vi "UpdateSequence.vi"(8 "error in":errorcluster, 10 "Cluster IN":T1, 11 "DataLogger in":refnum<class "DataLogger.lvclass">) -> (0 "error out":errorcluster, 2 "UpdateComplete":bool, 3 "Cluster OUT":T1)   [LabVIEW 2019, in "DataLogger.lvclass"]
doc: "Update Sequence"
uses:
  DataLogger.lvclass
  <vilib>/vision/Image Controls.llb/IMAQ Image.ctl
  Common/Controls/AllPartInfo.ctl
  Controls/LocalData_DL.ctl
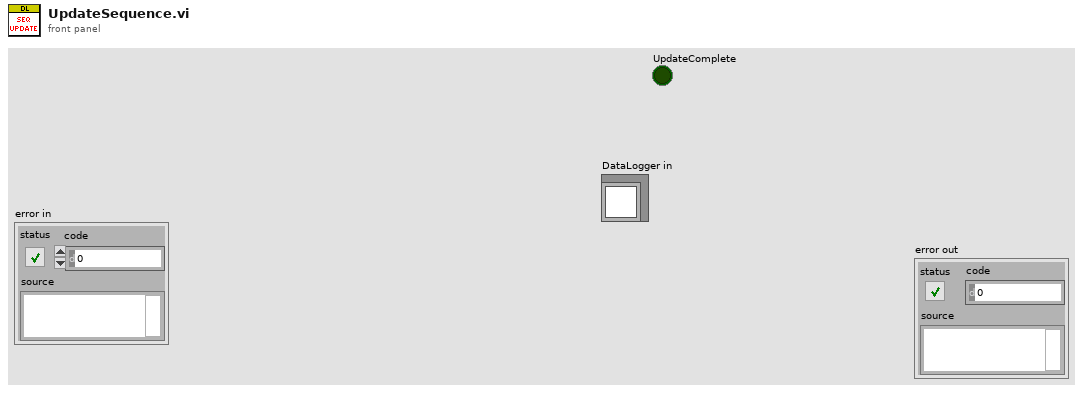
[diagram p1: front panel]
types:
  T1 = typedef "DataLogger.lvclass/LocalData_DL.ctl" = cluster{"Core":cluster{"Current VI Reference":refnum<vi>, "Close Panel on Exit?":bool}, "System Info":cluster{"System Name":string, "System ID":string, "Version":string, "Year":string, "Customer Details":cluster{"Customer Name":string, "Customer ID":string, "Location":string, "No of Shifts":u8, "Shift Details Array":cluster{"Name":string, "Timing":string}[]}, "Software Features":cluster{"IoT Enable":bool, "Datalogging Features":cluster{"Event Data":bool, "Measurement Data":bool, "Statistical Data":bool, "Reel Data":bool, "Failed Measurement Data":bool, "Failed Images":bool}, "IoT":cluster{"SMS Alert Enable":bool, "Email Alert Enable":bool}, "Popup Enable?":cluster{"Fail":bool, "Pause":bool, "Stop":bool}}}, "Part Info":cluster{"Part Name":string, "Rack ID":u8, "Initialize":bool, "StampingMc No":u64, "Operator Name":string, "ReelCount":u64, "TotalCount":u64, "Measurement Names Array":string[], "Measurement ID Array":u16[], "Spec Values Array":cluster{"LCL":dbl, "UCL":dbl, "LSL":dbl, "USL":dbl, "Nominal Value":dbl}[], "Camera Name Array":string[], "Measurement Enable/Disable Array":bool[], "Number of Measurements":i32}, "Fail Counter(For Event Details)":i32, "Event Details":cluster{"Event Name":string, "Event Time":string, "Event Reason":string, "Previous Event Name":string, "Previous Event Time":string}, "StatisticalInfo":string[][], "BatchInfo":cluster{"BatchPassCount":u64, "BatchFailCount":u64}, "Failure Details":cluster{"Fail Time Stamp":u64, "ControlPFArray":bool[], "SpecificationPFArray":dbl[], "Rack ID":u8, "Failed Image Array":T2[], "Fail Date":string, "Fail Time":string, "Fail Reason":string}, "SaveFailedImageCounter":i32, "AllPartInfoArray":T3, "Status":bool, "SpecValues(ForUpdate)":cluster{"LCL":dbl, "UCL":dbl, "LSL":dbl, "USL":dbl, "Nominal Value":dbl}, "AddSuccessfull":bool, "CurrentStateMessage":string, "IoTDetailsCounter":bool, "InitialUpdate":bool, "ResetUpdate":bool, "SetCounter":cluster{"MeasurementDetailsSetCounter":i32, "BatchDetailsSetCounter":i32, "FailureDetailsSetCounter":i32, "EventDetailsSetCounter":i32}, "IndexCounter":cluster{"MeasurementDetailsIndexCounter":i32, "BatchDetailsIndexCounter":i32, "FailureDetailsIndexCounter":i32, "EventDetailsIndexCounter":i32}, "Details2D":cluster{"MeasurementDetails(2D)":string[][], "BatchDetails(2D)":string[][], "FailureDetails(2D)":string[][], "EventDetails(2D)":string[][]}, "IDs":cluster{"Stamping McID":string, "Inspection McID":string, "BatchID":string, "FailID":string}, "Reel Info":cluster{"Reel No":u64, "Reel Start Time Stamp":u64}, "ExcelData":cluster{"StripPath":bool, "ReelCounterPerPart":i32, "FilePaths":cluster{"EventsFilePath":path, "FailFilePath":path, "ReelFilePath":path, "StatisticalFilePath":path}, "ExcelSheetCounterPerReel":cluster{"EventsSheetCounter":u32, "FailSheetCounter":u32, "StatisticalSheetCounter":u32, "ReelSheetCounter":u32}, "CreateNewExcel":cluster{"CreateNewEventsExcel":bool, "CreateNewFailExcel":bool, "CreateNewStatisticalExcel":bool, "CreateNewReelExcel":bool}, "RecordsInExcelCounter":cluster{"EventsRecordsCounter":u32, "FailRecordsCounter":u32, "ReelRecordsCounter":u32, "StatisticalRecordsCounter":u32}}, "SaveAck":cluster{"Loop1":bool, "Loop2":bool}, "Shift Statistical Info":cluster{"Shift Name":string, "Shift Timing":string, "Shift End Date":string, "Statistical Shift Data":cluster{"PartName":string, "MeasurementNames":string[], "Statistical Parameters":string[][]}[]}}
  T2 = typedef "IMAQ Image.ctl" = refnum<image>
  T3 = typedef "AllPartInfo.ctl" = cluster{"PartName":string, "NumberOfRacks":u8, "MeasurementIDsArray":u16[], "MeasurementNamesArray":string[], "SpecValuesArray":cluster{"LCL":dbl, "UCL":dbl, "LSL":dbl, "USL":dbl, "NominalValue":dbl}[]}[]
  T4 = cluster{"LCL":dbl, "UCL":dbl, "LSL":dbl, "USL":dbl, "NominalValue":dbl}[]
  T5 = cluster{"LCL":dbl, "UCL":dbl, "LSL":dbl, "USL":dbl, "Nominal Value":dbl}[]
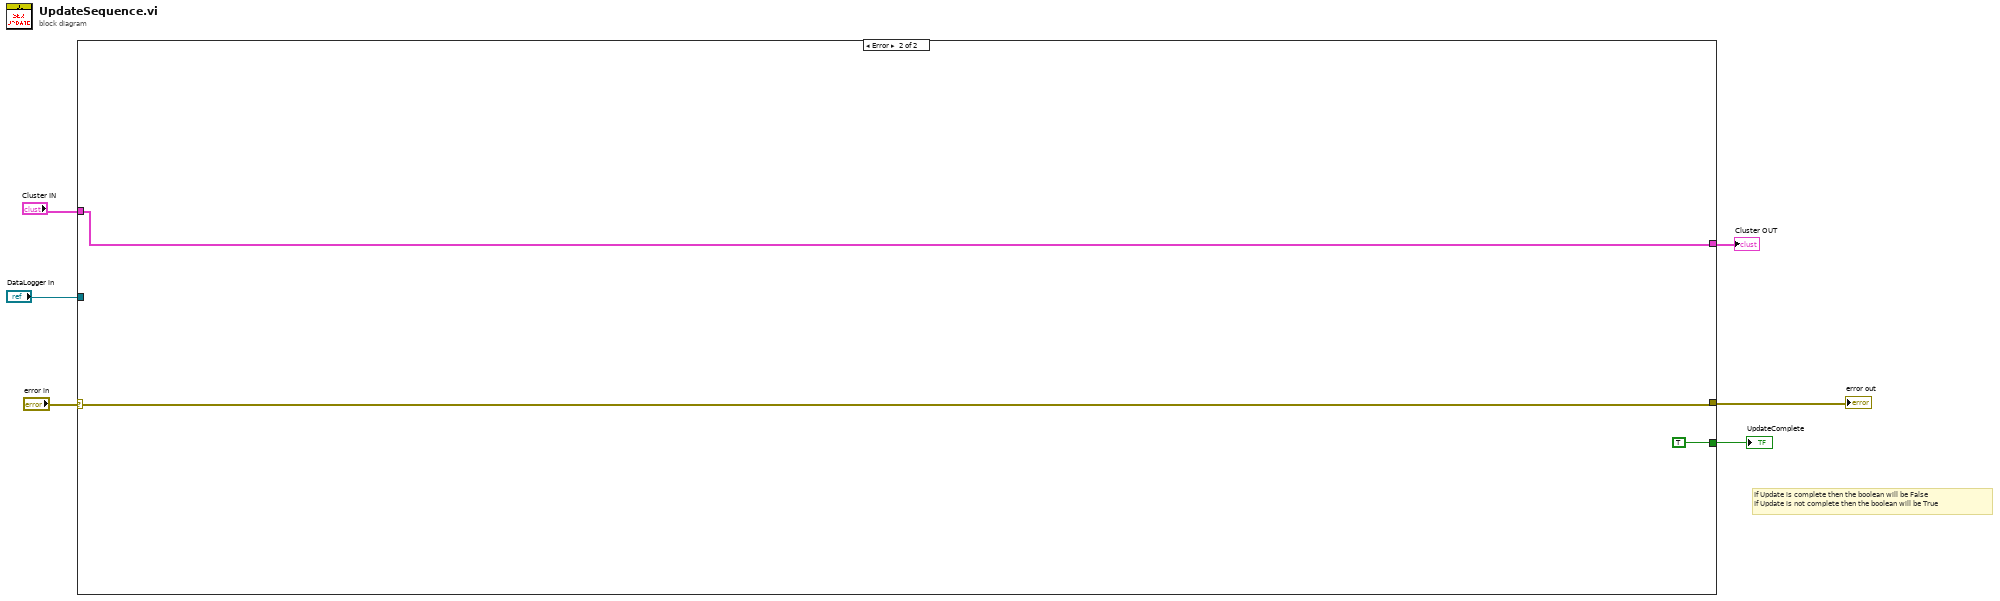
[diagram p0: block diagram]
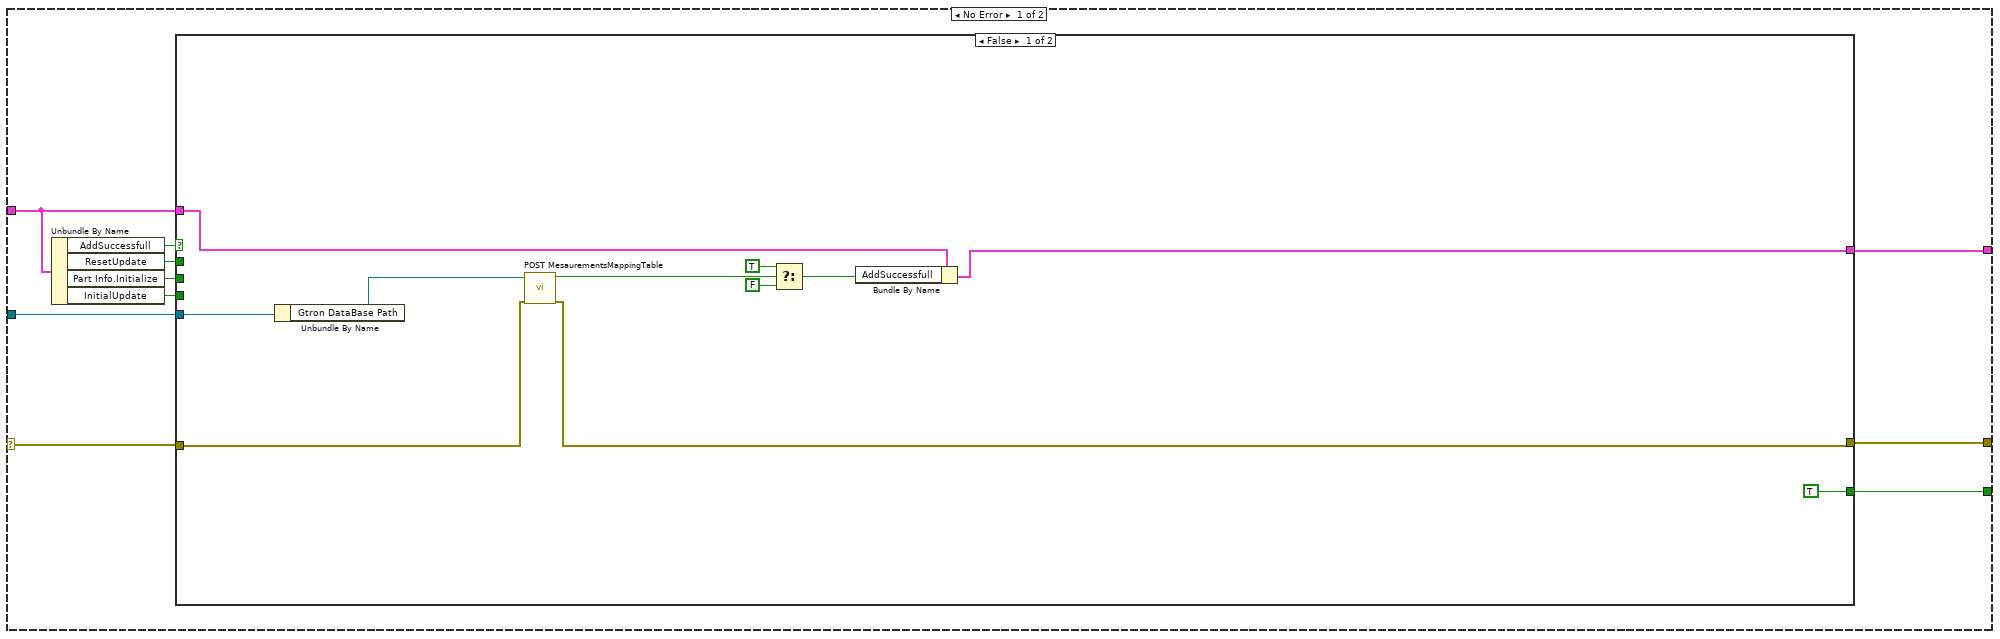
[diagram p2: hidden frame]
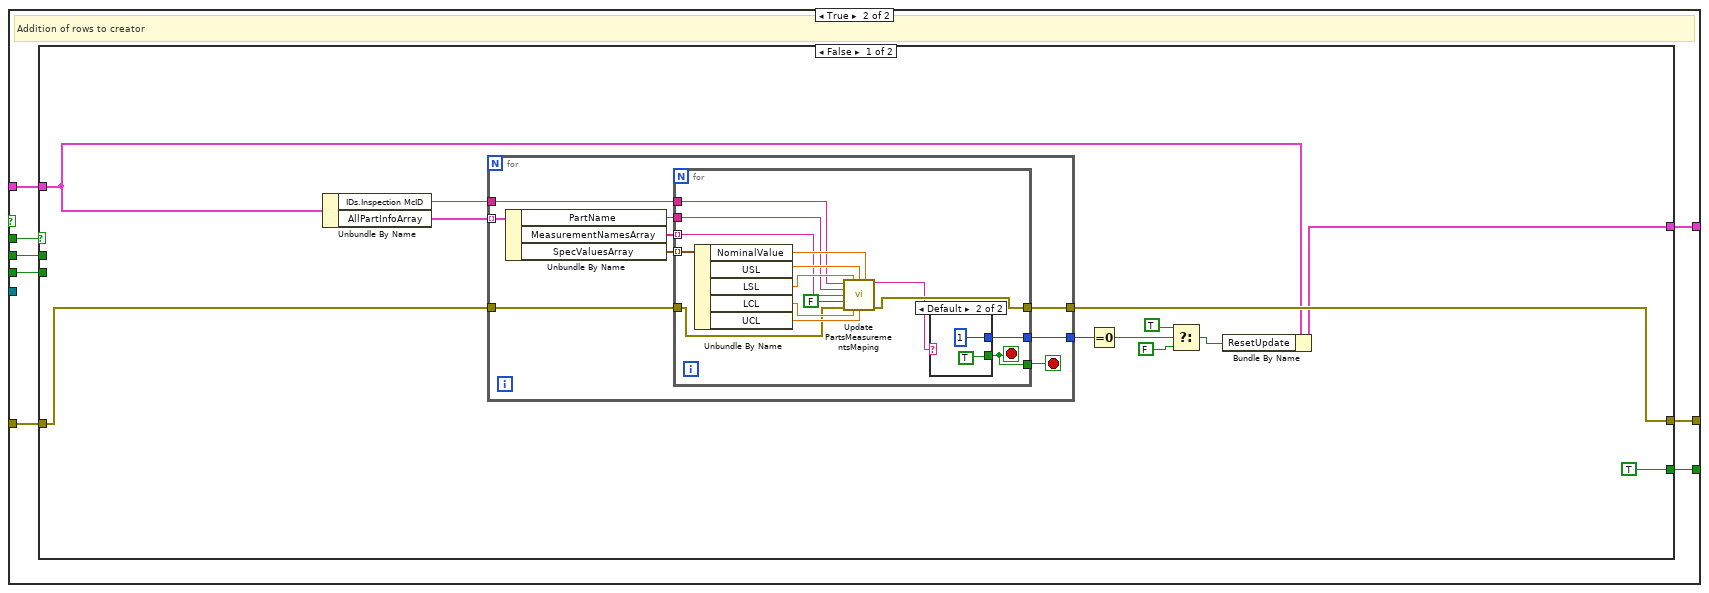
[diagram p3: hidden frame]
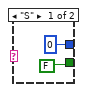
[diagram p4: hidden frame]
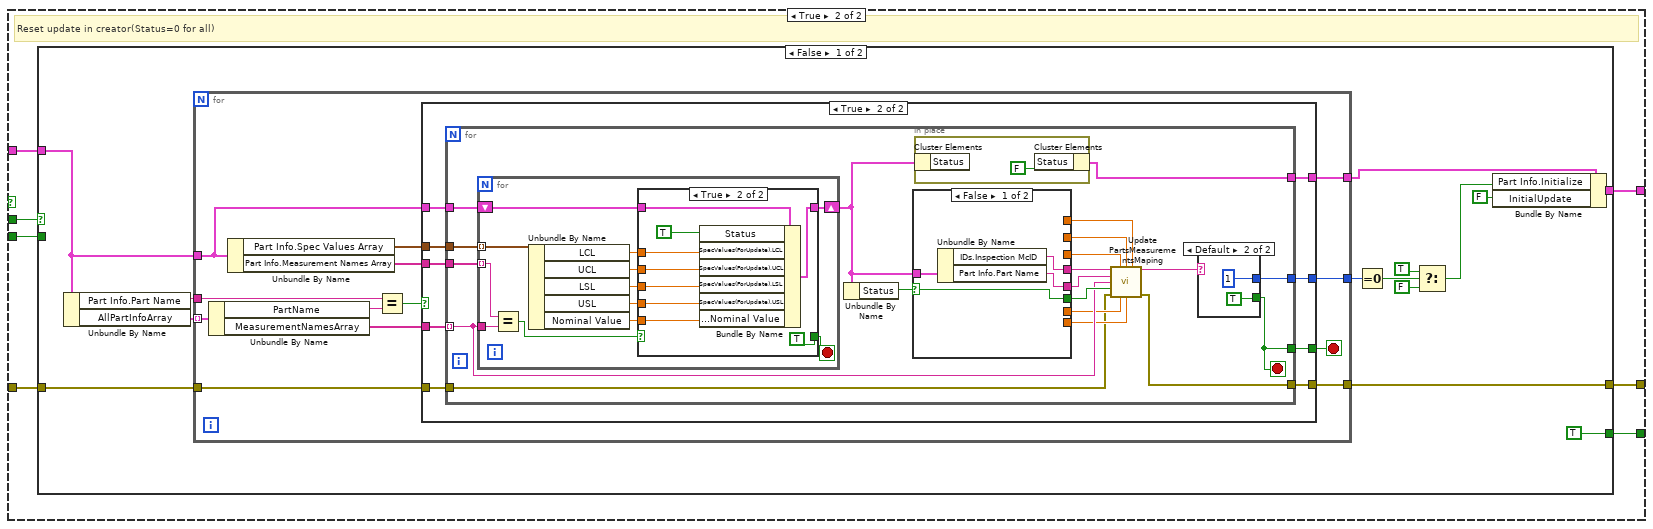
[diagram p5: hidden frame]
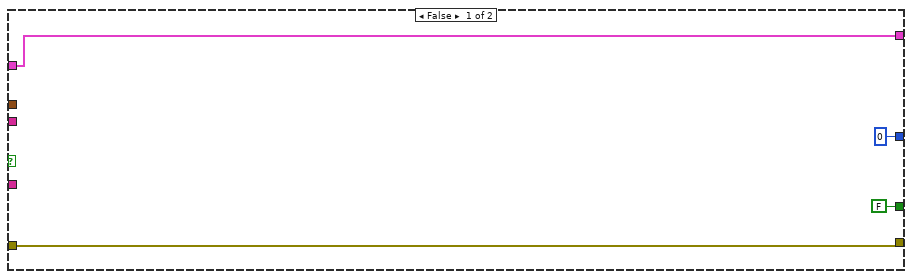
[diagram p6: hidden frame]
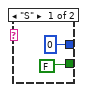
[diagram p7: hidden frame]
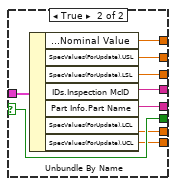
[diagram p8: hidden frame]
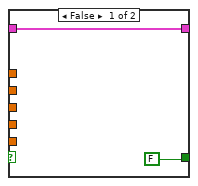
[diagram p9: hidden frame]
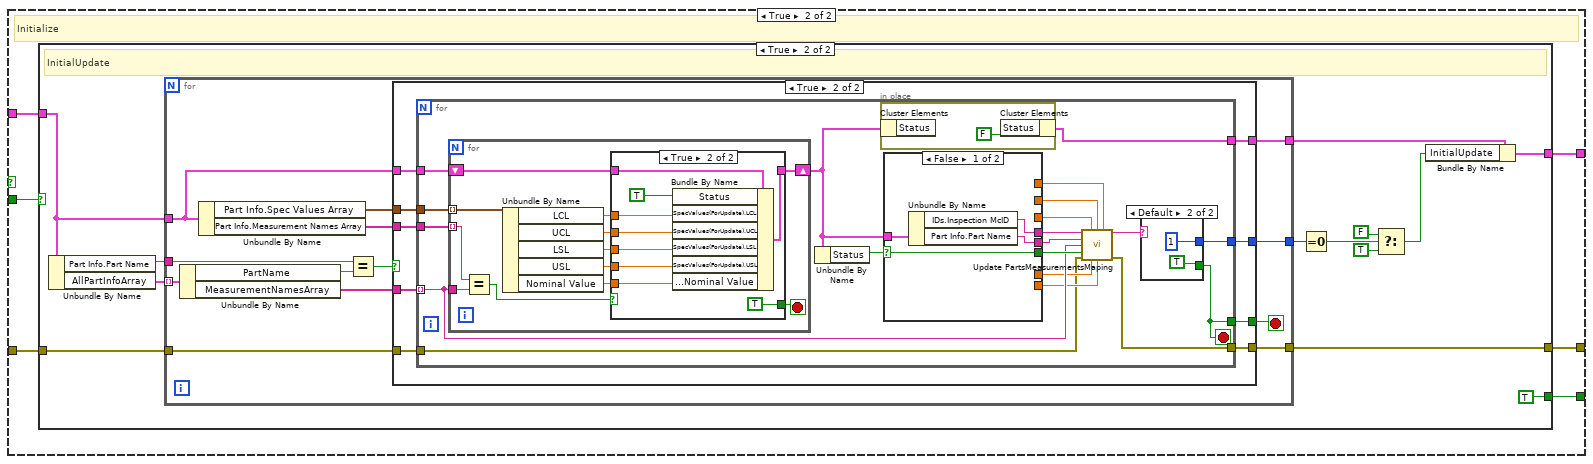
[diagram p10: hidden frame]
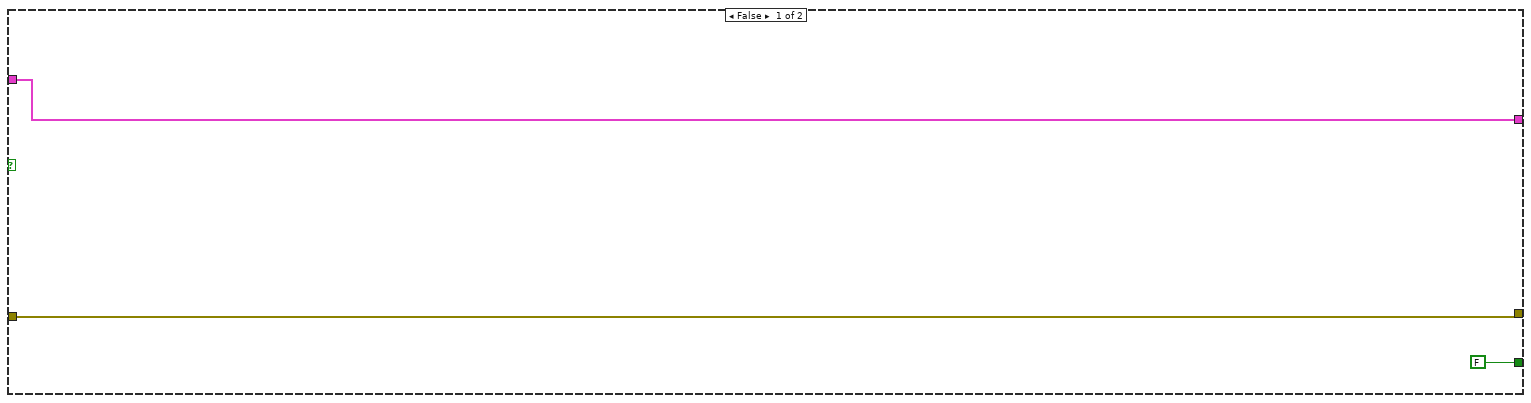
[diagram p11: hidden frame]
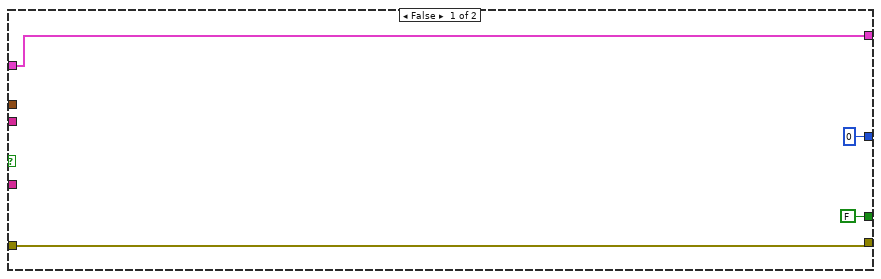
[diagram p12: hidden frame]
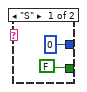
[diagram p13: hidden frame]
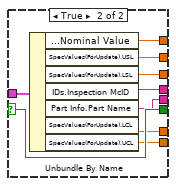
[diagram p14: hidden frame]
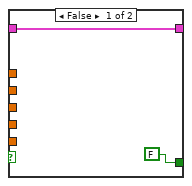
[diagram p15: hidden frame]
diagram:
  # "If Update is complete then the boolean will be False\nIf Update is not complete then the boolean will be True"
  n1 = case shown="Error" "error in" {
    selector: "error in" -> [w11 w295]
    tunnel: [w14 w295] -> w6
    tunnel: "DataLogger in" -> [w10 _]
    tunnel: "Cluster IN" -> [w9 w294]
    tunnel: [w8 w294] -> w2
    tunnel: [w7 TRUE] -> w1
    frame No Error {
      n2 = Unbundle By Name(w9) -> ("AddSuccessfull"=w15:bool, "ResetUpdate"=w16:bool, "Part Info.Initialize"=w13:bool, "InitialUpdate"=w12:bool)
      n3 = case shown="False" w15 {
        tunnel: w9 -> [w24 w35]
        tunnel: w13 -> [_ w34]
        tunnel: [w23 w33] -> w8
        tunnel: w11 -> [w19 w32]
        tunnel: [w18 w31] -> w14
        tunnel: w10 -> [w21 _]
        tunnel: w12 -> [_ w30]
        tunnel: w16 -> [_ w29]
        tunnel: [TRUE w28] -> w7
        frame False {
          n4 = Unbundle By Name(w21) -> ("Gtron DataBase Path"=w20:path)
          n5 = call "POST MesaurementsMappingTable.vi"("error in"=w19, "GTron in"=w20) -> ("error out"=w18:errorcluster, "DB is Empty?"=w22:bool)  [unwired: 8 in]
          n6 = Select(t=TRUE, s=w22, f=FALSE) -> (s? t:f=w25:bool)
          n7 = Bundle By Name(cluster=w24, "AddSuccessfull"=w25) -> (w23:T1)
        }
        frame True {
          # "Addition of rows to creator"
          n8 = case shown="False" w29 {
            tunnel: w35 -> [w40 w82]
            tunnel: w34 -> [_ w81]
            tunnel: [w41 w80] -> w33
            tunnel: w32 -> [w43 w79]
            tunnel: [w42 w78] -> w31
            tunnel: w30 -> [_ w77]
            tunnel: [TRUE w76] -> w28
            frame False {
              n9 = Unbundle By Name(w40) -> ("IDs.Inspection McID"=w39:string, "AllPartInfoArray"=w47:T3)
              n10 = for {
                tunnel: w47 -> [w56] mode=indexing
                tunnel: w43 -> [w52]
                tunnel: [w51] -> w42
                tunnel: [w49] -> w37
                tunnel: w39 -> [w48]
                stop <- w50 stop-if-true
                n11 = Unbundle By Name(w56) -> ("PartName"=w54:string, "MeasurementNamesArray"=w55:string[], "SpecValuesArray"=w53:T4)
                n12 = for {
                  tunnel: w55 -> [w66] mode=indexing
                  tunnel: w54 -> [w67]
                  tunnel: w53 -> [w71] mode=indexing
                  tunnel: w52 -> [w62]
                  tunnel: [w61] -> w51
                  tunnel: [w58] -> w50
                  tunnel: [w59] -> w49
                  tunnel: w48 -> [w57]
                  stop <- w58 stop-if-true
                  n13 = Unbundle By Name(w71) -> ("NominalValue"=w70:dbl, "USL"=w69:dbl, "LSL"=w68:dbl, "LCL"=w64:dbl, "UCL"=w63:dbl)
                  n14 = call "Update PartsMeasurementsMaping.vi"("InspectionMcId"=w57, "NewLSL"=w68, "NewUSL"=w69, "NewNominalValue"=w70, "PartName"=w67, "MeasurementName"=w66, "Status1"=FALSE ("Status"), "error in"=w62, "NewLCL"=w64, "NewUCL"=w63) -> ("Status"=w60:string, "error out"=w61:errorcluster)  [unwired: 4 in]
                  n15 = case shown="Default" w60 {
                    tunnel: [0 1] -> w59
                    tunnel: [FALSE TRUE] -> w58
                    frame "S" {
                    }
                    frame Default {
                    }
                  }
                }
              }
              n16 = Equal To 0?(x=w37) -> (x = 0?=w38:bool)
              n17 = Select(t=TRUE, s=w38, f=FALSE) -> (s? t:f=w44:bool)
              n18 = Bundle By Name(cluster=w40, "ResetUpdate"=w44) -> (w41:T1)
            }
            frame True {
              # "Reset update in creator(Status=0 for all)"
              n19 = case shown="False" w81 {
                tunnel: w82 -> [w93 w188]
                tunnel: [w94 w189] -> w80
                tunnel: w79 -> [w91 w187]
                tunnel: [w90 w186] -> w78
                tunnel: w77 -> [_ w185]
                tunnel: [TRUE w184] -> w76
                frame False {
                  n20 = Unbundle By Name(w93) -> ("Part Info.Part Name"=w95:string, "AllPartInfoArray"=w96:T3)
                  n21 = for {
                    tunnel: w96 -> [w109] mode=indexing
                    tunnel: w95 -> [w107]
                    tunnel: w93 -> [w102]
                    tunnel: [w101] -> w92
                    tunnel: w91 -> [w100]
                    tunnel: [w99] -> w90
                    tunnel: [w97] -> w85
                    stop <- w98 stop-if-true
                    n22 = Unbundle By Name(w109) -> ("PartName"=w108:string, "MeasurementNamesArray"=w105:string[])
                    n23 = Unbundle By Name(w102) -> ("Part Info.Spec Values Array"=w104:T5, "Part Info.Measurement Names Array"=w103:string[])
                    n24 = Equal?(x=w107, y=w108) -> (x = y?=w106:bool)
                    n25 = case shown="True" w106 {
                      tunnel: w105 -> [_ w122]
                      tunnel: w104 -> [_ w121]
                      tunnel: w103 -> [_ w120]
                      tunnel: w102 -> [w113 w119]
                      tunnel: [w113 w118] -> w101
                      tunnel: w100 -> [w112 w117]
                      tunnel: [w112 w116] -> w99
                      tunnel: [FALSE w115] -> w98
                      tunnel: [0 w114] -> w97
                      frame False {
                      }
                      frame True {
                        n26 = for {
                          tunnel: w122 -> [w137] mode=indexing
                          tunnel: w121 -> [w142]
                          tunnel: w120 -> [w141]
                          tunnel: w119 -> [w140]
                          tunnel: [w123] -> w118
                          tunnel: w117 -> [w129]
                          tunnel: [w128] -> w116
                          tunnel: [w126] -> w115
                          tunnel: [w125] -> w114
                          stop <- w126 stop-if-true
                          n27 = for {
                            tunnel: w142 -> [w167] mode=indexing
                            tunnel: w141 -> [w172] mode=indexing
                            tunnel: w137 -> [w171]
                            shift-right: [w168] -> w124
                            shift-left: w140 -> [w170]
                            stop <- w161 stop-if-true
                            n28 = Equal?(x=w172, y=w171) -> (x = y?=w169:bool)
                            n29 = Unbundle By Name(w167) -> ("LCL"=w162:dbl, "UCL"=w163:dbl, "LSL"=w164:dbl, "USL"=w165:dbl, "Nominal Value"=w166:dbl)
                            n30 = case shown="True" w169 {
                              tunnel: w170 -> [w174 w183]
                              tunnel: [w174 w181] -> w168
                              tunnel: w166 -> [_ w180]
                              tunnel: w165 -> [_ w179]
                              tunnel: w164 -> [_ w178]
                              tunnel: w163 -> [_ w177]
                              tunnel: w162 -> [_ w176]
                              tunnel: [FALSE TRUE] -> w161
                              frame False {
                              }
                              frame True {
                                n31 = Bundle By Name(cluster=w183, "Status"=TRUE, "SpecValues(ForUpdate).LCL"=w176, "SpecValues(ForUpdate).UCL"=w177, "SpecValues(ForUpdate).LSL"=w178, "SpecValues(ForUpdate).USL"=w179, "SpecValues(ForUpdate).Nominal Value"=w180) -> (w181:T1)
                              }
                            }
                          }
                          n32 = Unbundle By Name(w124) -> ("Status"=w139:bool)
                          n33 = case shown="False" w139 {
                            selector: w139 -> [w151 w159]
                            tunnel: w124 -> [w150 w160]
                            tunnel: [w151 w159] -> w138
                            tunnel: [_ w158] -> w136
                            tunnel: [_ w157] -> w135
                            tunnel: [_ w156] -> w134
                            tunnel: [_ w155] -> w133
                            tunnel: [_ w154] -> w132
                            tunnel: [w149 w153] -> w131
                            tunnel: [w148 w152] -> w130
                            frame False {
                              n34 = Unbundle By Name(w150) -> ("IDs.Inspection McID"=w149:string, "Part Info.Part Name"=w148:string)
                            }
                            frame True {
                              n35 = Unbundle By Name(w160) -> ("SpecValues(ForUpdate).Nominal Value"=w158:dbl, "SpecValues(ForUpdate).USL"=w157:dbl, "SpecValues(ForUpdate).LSL"=w156:dbl, "IDs.Inspection McID"=w153:string, "Part Info.Part Name"=w152:string, "SpecValues(ForUpdate).LCL"=w154:dbl, "SpecValues(ForUpdate).UCL"=w155:dbl)
                            }
                          }
                          n36 = in-place {
                            n37 = in-place-cluster #1(w124) -> ()  [unwired: 1 out]
                            n38 = in-place-cluster #1("Status"=FALSE) -> (w123:T1)
                          }
                          n39 = call "Update PartsMeasurementsMaping.vi"("InspectionMcId"=w131, "NewLSL"=w134, "NewUSL"=w135, "NewNominalValue"=w136, "PartName"=w130, "MeasurementName"=w137, "Status1"=w138, "error in"=w129, "NewLCL"=w132, "NewUCL"=w133) -> ("Status"=w127:string, "error out"=w128:errorcluster)  [unwired: 4 in]
                          n40 = case shown="Default" w127 {
                            tunnel: [0 1] -> w125
                            tunnel: [FALSE TRUE] -> w126
                            frame "S" {
                            }
                            frame Default {
                            }
                          }
                        }
                      }
                    }
                  }
                  n41 = Equal To 0?(x=w85) -> (x = 0?=w84:bool)
                  n42 = Select(t=TRUE, s=w84, f=FALSE) -> (s? t:f=w86:bool)
                  n43 = Bundle By Name(cluster=w92, "Part Info.Initialize"=w86, "InitialUpdate"=FALSE ("Reinitialize?")) -> (w94:T1)
                }
                frame True {
                  # "Initialize"
                  n44 = case shown="True" w185 {
                    tunnel: [w192 w203] -> w189
                    tunnel: w188 -> [w192 w202]
                    tunnel: w187 -> [w191 w200]
                    tunnel: [w191 w199] -> w186
                    tunnel: [FALSE TRUE] -> w184
                    frame False {
                    }
                    frame True {
                      # "InitialUpdate"
                      n45 = Unbundle By Name(w202) -> ("Part Info.Part Name"=w204:string, "AllPartInfoArray"=w205:T3)
                      n46 = for {
                        tunnel: w205 -> [w218] mode=indexing
                        tunnel: w204 -> [w216]
                        tunnel: w202 -> [w211]
                        tunnel: [w210] -> w201
                        tunnel: w200 -> [w209]
                        tunnel: [w208] -> w199
                        tunnel: [w206] -> w194
                        stop <- w207 stop-if-true
                        n47 = Unbundle By Name(w218) -> ("PartName"=w217:string, "MeasurementNamesArray"=w214:string[])
                        n48 = Unbundle By Name(w211) -> ("Part Info.Spec Values Array"=w213:T5, "Part Info.Measurement Names Array"=w212:string[])
                        n49 = Equal?(x=w216, y=w217) -> (x = y?=w215:bool)
                        n50 = case shown="True" w215 {
                          tunnel: w214 -> [_ w231]
                          tunnel: w213 -> [_ w230]
                          tunnel: w212 -> [_ w229]
                          tunnel: w211 -> [w222 w228]
                          tunnel: [w222 w227] -> w210
                          tunnel: w209 -> [w221 w226]
                          tunnel: [w221 w225] -> w208
                          tunnel: [FALSE w224] -> w207
                          tunnel: [0 w223] -> w206
                          frame False {
                          }
                          frame True {
                            n51 = for {
                              tunnel: w231 -> [w246] mode=indexing
                              tunnel: w230 -> [w251]
                              tunnel: w229 -> [w250]
                              tunnel: w228 -> [w249]
                              tunnel: [w232] -> w227
                              tunnel: w226 -> [w238]
                              tunnel: [w237] -> w225
                              tunnel: [w235] -> w224
                              tunnel: [w234] -> w223
                              stop <- w235 stop-if-true
                              n52 = for {
                                tunnel: w251 -> [w276] mode=indexing
                                tunnel: w250 -> [w281] mode=indexing
                                tunnel: w246 -> [w280]
                                shift-right: [w277] -> w233
                                shift-left: w249 -> [w279]
                                stop <- w270 stop-if-true
                                n53 = Equal?(x=w281, y=w280) -> (x = y?=w278:bool)
                                n54 = Unbundle By Name(w276) -> ("LCL"=w271:dbl, "UCL"=w272:dbl, "LSL"=w273:dbl, "USL"=w274:dbl, "Nominal Value"=w275:dbl)
                                n55 = case shown="True" w278 {
                                tunnel: w279 -> [w283 w292]
                                tunnel: [w283 w290] -> w277
                                tunnel: w275 -> [_ w289]
                                tunnel: w274 -> [_ w288]
                                tunnel: w273 -> [_ w287]
                                tunnel: w272 -> [_ w286]
                                tunnel: w271 -> [_ w285]
                                tunnel: [FALSE TRUE] -> w270
                                frame False {
                                }
                                frame True {
                                n56 = Bundle By Name(cluster=w292, "Status"=TRUE, "SpecValues(ForUpdate).LCL"=w285, "SpecValues(ForUpdate).UCL"=w286, "SpecValues(ForUpdate).LSL"=w287, "SpecValues(ForUpdate).USL"=w288, "SpecValues(ForUpdate).Nominal Value"=w289) -> (w290:T1)
                                }
                                }
                              }
                              n57 = Unbundle By Name(w233) -> ("Status"=w248:bool)
                              n58 = in-place {
                                n59 = in-place-cluster #2(w233) -> ()  [unwired: 1 out]
                                n60 = in-place-cluster #2("Status"=FALSE) -> (w232:T1)
                              }
                              n61 = case shown="False" w248 {
                                selector: w248 -> [w260 w268]
                                tunnel: w233 -> [w259 w269]
                                tunnel: [w260 w268] -> w247
                                tunnel: [_ w267] -> w245
                                tunnel: [_ w266] -> w244
                                tunnel: [_ w265] -> w243
                                tunnel: [_ w264] -> w242
                                tunnel: [_ w263] -> w241
                                tunnel: [w258 w262] -> w240
                                tunnel: [w257 w261] -> w239
                                frame False {
                                n62 = Unbundle By Name(w259) -> ("IDs.Inspection McID"=w258:string, "Part Info.Part Name"=w257:string)
                                }
                                frame True {
                                n63 = Unbundle By Name(w269) -> ("SpecValues(ForUpdate).Nominal Value"=w267:dbl, "SpecValues(ForUpdate).USL"=w266:dbl, "SpecValues(ForUpdate).LSL"=w265:dbl, "IDs.Inspection McID"=w262:string, "Part Info.Part Name"=w261:string, "SpecValues(ForUpdate).LCL"=w263:dbl, "SpecValues(ForUpdate).UCL"=w264:dbl)
                                }
                              }
                              n64 = call "Update PartsMeasurementsMaping.vi"("InspectionMcId"=w240, "NewLSL"=w243, "NewUSL"=w244, "NewNominalValue"=w245, "PartName"=w239, "MeasurementName"=w246, "Status1"=w247, "error in"=w238, "NewLCL"=w241, "NewUCL"=w242) -> ("Status"=w236:string, "error out"=w237:errorcluster)  [unwired: 4 in]
                              n65 = case shown="Default" w236 {
                                tunnel: [0 1] -> w234
                                tunnel: [FALSE TRUE] -> w235
                                frame "S" {
                                }
                                frame Default {
                                }
                              }
                            }
                          }
                        }
                      }
                      n66 = Equal To 0?(x=w194) -> (x = 0?=w195:bool)
                      n67 = Select(t=FALSE, s=w195, f=TRUE) -> (s? t:f=w196:bool)
                      n68 = Bundle By Name(cluster=w201, "InitialUpdate"=w196) -> (w203:T1)
                    }
                  }
                }
              }
            }
          }
        }
      }
    }
    frame Error {
    }
  }
  "error out" <- w6
  "Cluster OUT" <- w2
  "UpdateComplete" <- w1
